vi "_XNET Convert Time U64 to LV.vi"(3 "Time U64":u64) -> (1 "Time LV":timestamp)   [LabVIEW 2018]
uses:
  nixlvapi.dll
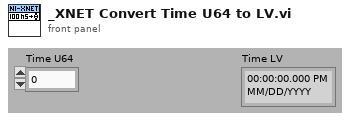
[diagram p1: front panel]
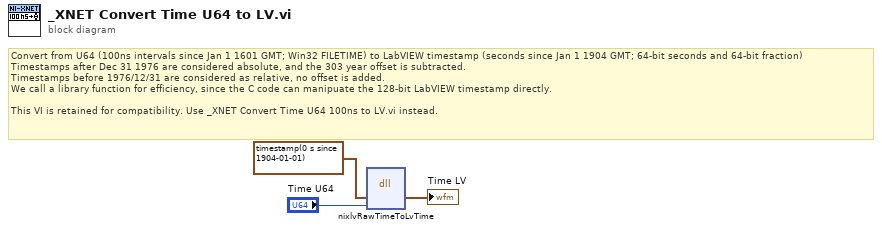
[diagram p0: block diagram]
diagram:
  # "Convert from U64 (100ns intervals since Jan 1 1601 GMT; Win32 FILETIME) to LabVIEW timestamp (seconds since Jan 1 1904 GMT; 64-bit seconds and 64-bit fraction)\nTimestamps after Dec 31 1976 are considered absolute, and the 303 year offset is subtracted.\nTimestamps before 1976/12/31 are considered as relative, no offset is added.\nWe call a library function for efficiency, since the C code can manipuate the 128-bit LabVIEW timestamp directly.\n\nThis VI is retained for compatibility. Use _XNET Convert Time U64 100ns to LV.vi instead."
  n1 = dll-call lib="nixlvapi.*" fn="nixlvRawTimeToLvTime" label="Call Library"("lvTime"=timestamp(0 s since 1904-01-01) ("Time LV"), "rawTime"="Time U64") -> ("lvTime"=→"Time LV":timestamp)  [unwired: 4 in, 3 out]
